vi "MobileTest_RunTest.vi"() -> ()   [LabVIEW 2019]
uses:
  Public/Documents/National Instruments/TestStand 2019 (64-bit)/Examples/Demos/Mobile Device Test/LabVIEW/Source/Support/Wifi Test Modes.ctl
panel:
  out "Image Report String":string
  out "QAM Data Transmitted":cluster{dbl[], dbl[]}(graph)
  out "Error Out":errorcluster
  out "UUT String Received":string
  out "QAM Data Received":cluster{dbl[], dbl[]}(graph)
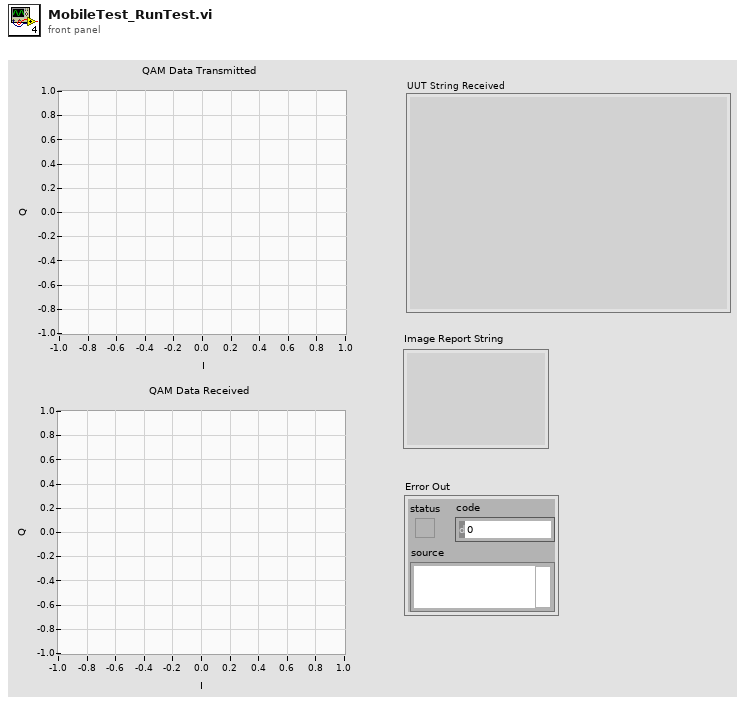
[diagram p1: front panel]
types:
  T1 = typedef "Wifi Test Modes.ctl" = enum16{"802.11b/g/n (QAM-16)", "LTE (QAM-64)", "802.11ac (QAM-256)"}
  T2 = cluster{"QAM Data Transmitted":cluster{dbl[], dbl[]}, "QAM Data Received":cluster{dbl[], dbl[]}, "symbol map 16 QAM":cdb[], "Mode":T1}
  T3 = cluster{"Output String":string, "Report String":string}
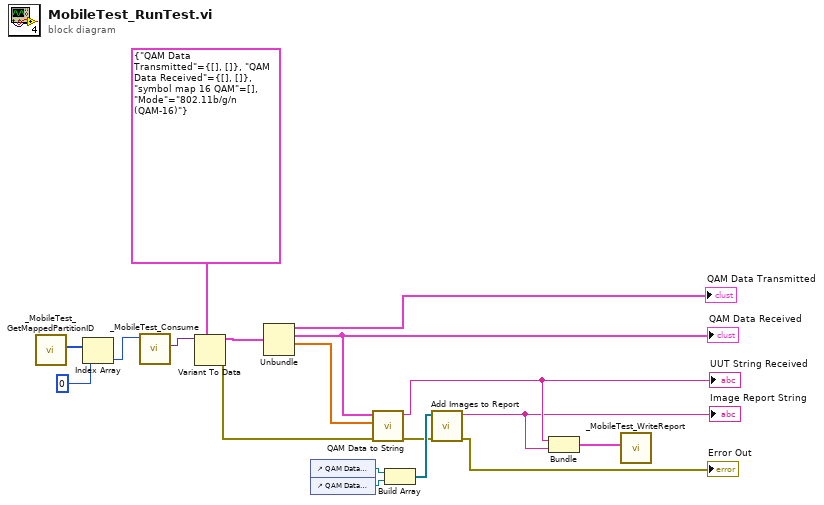
[diagram p0: block diagram]
diagram:
  n1 = call "_MobileTest_GetMappedPartitionID.vi"() -> ("ID"=w14:u32[])  [unwired: 11 in]
  n2 = Index Array(array=w14, index=0) -> (element=w9:u32)
  n3 = call "_MobileTest_Consume.vi"("ID"=w9) -> ("Data"=w8:variant)  [unwired: 8 in]
  n4 = Variant To Data(type=T2 {"QAM Data Transmitted"={[], []}, "QAM Data Received"={[], []}, "symbol map 16 QAM"=[], "Mode"=enum."802.11b/g/n (QAM-16)"} ("output cluster"), Variant=w8) -> (data=w6:T2, error out=w5:errorcluster)  [unwired: 1 in]
  n5 = Unbundle(w6) -> ("QAM Data Transmitted"=→"QAM Data Transmitted":cluster{dbl[], dbl[]}, "QAM Data Received"=w1:cluster{dbl[], dbl[]}, "symbol map 16 QAM"=w2:cdb[])  [unwired: 1 out]
  "QAM Data Received" <- w1
  n6 = control-ref of="QAM Data Received"() -> (w18:refnum<vi>)
  n7 = control-ref of="QAM Data Transmitted"() -> (w17:refnum<vi>)
  n8 = call "QAM Data to String.vi"("error in (no error)"=w5, "symbol map 16 QAM"=w2, "QAM Data Out"=w1) -> ("error out"=w15:errorcluster, "Output String"=w12:string)  [unwired: 7 in]
  "UUT String Received" <- w12
  n9 = Build Array(w18, w17) -> (w16:refnum<vi>[])
  n10 = call "Add Images to Report.vi"("error in (no error)"=w15, "Control References"=w16) -> ("error out"=→"Error Out":errorcluster, "Report String"=w11:string)  [unwired: 8 in]
  "Image Report String" <- w11
  n11 = Bundle("Output String"=w12, "Report String"=w11) -> (w10:T3)  [unwired: 1 in]
  n12 = call "_MobileTest_WriteReport.vi"("Data"=w10) -> ()  [unwired: 8 in]
